vi "Channel(4800).vi"(7 "Выборка\nс передатчика":cdb format="%#.6g") -> (8 "Выборка \nс канала":cdb)   [LabVIEW 2013]
uses:
  <vilib>/ptbypt/NI_PtbyPt.lvlib
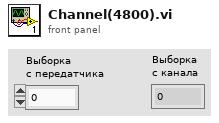
[diagram p1: front panel]
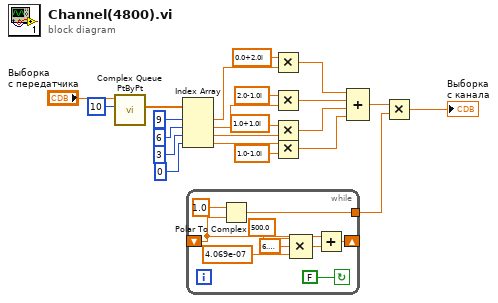
[diagram p0: block diagram]
diagram:
  n1 = call <vilib>:"Complex Queue PtByPt.vi"("sample length"=10, "input data point"="Выборка\nс передатчика") -> ("Current Queue"=w20:cdb[])  [unwired: 5 in, 4 out]
  n2 = Index Array(array=w20, index #1=9 ("index"), index #2=6 ("index"), index #3=3 ("index"), index #4=0 ("index")) -> (element #1=w15:cdb, element #2=w14:cdb, element #3=w13:cdb, element #4=w12:cdb)
  n3 = while {
    shift-right: [w26] -> _
    shift-left: _ -> [w25]
    tunnel: [w23] -> w5
    stop <- FALSE continue-if-true
    n4 = Polar To Complex(1:w25, 2:1.0 ("r")) -> (0:w23:cdb)
    n5 = Compound Arithmetic op=MULTIPLY(500.0, 6.283185307179586, 4.069e-07 ("value")) -> (w27:dbl)
    n6 = Add(x=w25, y=w27) -> (x+y=w26:dbl)
  }
  n7 = Multiply(x=cdb 0.0+2.0i, y=w15) -> (x*y=w7:cdb)
  n8 = Multiply(x=cdb 2.0-1.0i, y=w14) -> (x*y=w3:cdb)
  n9 = Multiply(x=cdb 1.0+1.0i, y=w13) -> (x*y=w2:cdb)
  n10 = Multiply(x=w12, y=cdb 1.0-1.0i) -> (x*y=w1:cdb)
  n11 = Compound Arithmetic op=ADD(w7, w3, w2, w1) -> (w6:cdb)
  n12 = Multiply(x=w6, y=w5) -> (x*y=→"Выборка \nс канала":cdb)
